vi "Enum from Value.vi"(10 "Value":i32) -> (2 "Enumeration":T1)   [LabVIEW 2020, in "AckNackResult.lvlib"]
uses:
  AckNackResult.lvlib
  Enumeration.ctl
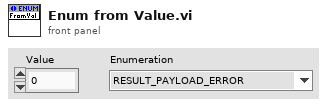
[diagram p1: front panel]
types:
  T1 = typedef "AckNackResult.lvlib/Enumeration.ctl" = enum16{"RESULT_PAYLOAD_ERROR", "RESULT_UNEXPECTED_TYPE", "RESULT_EXPIRED", "RESULT_OUTOFSEQUENCE", "RESULT_DISALLOWED", "RESULT_INVALIDTASK", "RESULT_INVALIDTARGET", "RESULT_UNKNOWN", "RESULT_ACK"}
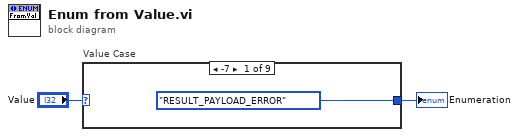
[diagram p0: block diagram]
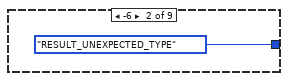
[diagram p2: hidden frame]
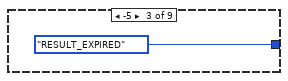
[diagram p3: hidden frame]
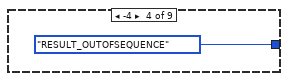
[diagram p4: hidden frame]
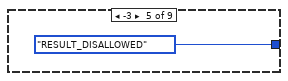
[diagram p5: hidden frame]
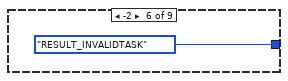
[diagram p6: hidden frame]
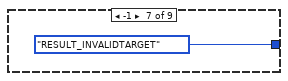
[diagram p7: hidden frame]
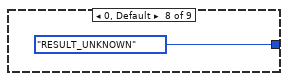
[diagram p8: hidden frame]
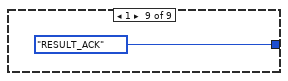
[diagram p9: hidden frame]
diagram:
  n1 = case "Value Case" shown="-7" "Value" {
    tunnel: [Enumeration."RESULT_PAYLOAD_ERROR" ("Enumeration") Enumeration."RESULT_UNEXPECTED_TYPE" ("Enumeration") Enumeration."RESULT_EXPIRED" ("Enumeration") Enumeration."RESULT_OUTOFSEQUENCE" ("Enumeration") Enumeration."RESULT_DISALLOWED" ("Enumeration") Enumeration."RESULT_INVALIDTASK" ("Enumeration") Enumeration."RESULT_INVALIDTARGET" ("Enumeration") Enumeration."RESULT_UNKNOWN" ("Enumeration") Enumeration."RESULT_ACK" ("Enumeration")] -> w1
    frame -7 {
    }
    frame -6 {
    }
    frame -5 {
    }
    frame -4 {
    }
    frame -3 {
    }
    frame -2 {
    }
    frame -1 {
    }
    frame 0, Default {
    }
    frame 1 {
    }
  }
  "Enumeration" <- w1
